vi "사인파형(subVI).vi"() -> (0 "웨이브폼 그래프":dbl[](graph), 1 "경로 출력":path)   [LabVIEW 2014]
uses:
  <vilib>/Utility/file.llb/Write To Spreadsheet File (DBL).vi
  <vilib>/Analysis/NI_AALBase.lvlib
panel:
  in  "취소 버튼":bool
  in  "확인 버튼":bool
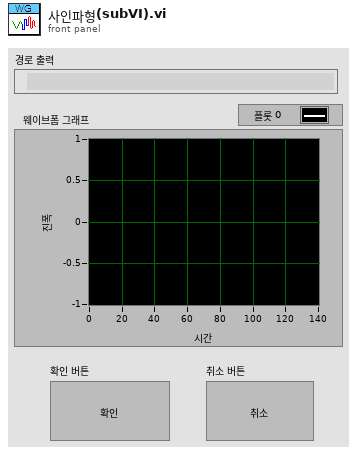
[diagram p1: front panel]
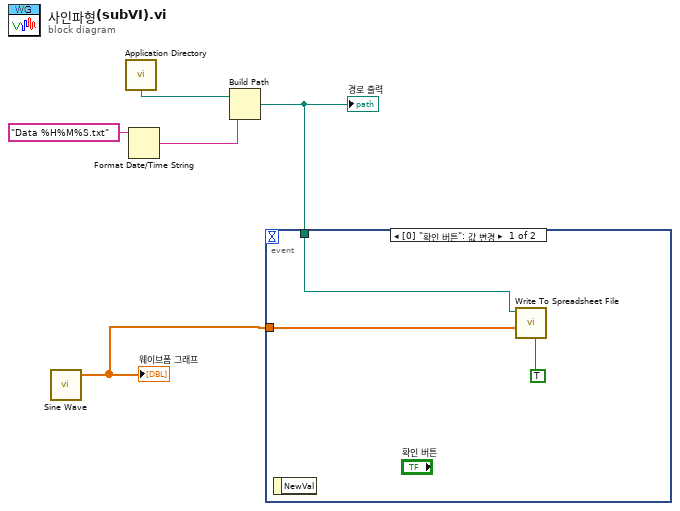
[diagram p0: block diagram]
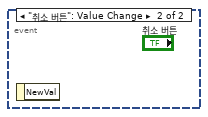
[diagram p2: hidden frame]
diagram:
  n1 = call <vilib>:"Sine Wave.vi"() -> ("sine wave"=w5:dbl[])  [unwired: 5 in, 2 out]
  "웨이브폼 그래프" <- w5
  n2 = call <vilib>:"Application Directory.vi"() -> ("Application Directory"=w3:path)
  n3 = Format Date/Time String(time format string (%c)="Data %H%M%S.txt" ("시간 포맷 문자열 (%c)")) -> (date/time string=w2:string)  [unwired: 2 in]
  n4 = Build Path(base path=w3, name or relative path=w2) -> (appended path=w1:path)
  "경로 출력" <- w1
  n5 = event shown="[0] \"확인 버튼\": 값 변경" {
    selector: _ -> [_ _]
    dyn-events: _ -> [_ _]
    timeout: _ -> [_ _]
    tunnel: w5 -> [w8 _]
    tunnel: w1 -> [w6 _]
    event "확인 버튼": Value Change {
      n6 = event-data() -> ()  [unwired: 1 in, 1 out]
      n7 = call-poly <vilib>:"Write To Spreadsheet File.vi"("transpose? (no:F)"=TRUE, "1D data"=w8, "file path (dialog if empty)"=w6) -> ()  [unwired: 5 in, 1 out]
    }
    event "취소 버튼": Value Change {
      n8 = event-data() -> ()  [unwired: 1 in, 1 out]
    }
  }
